vi "TCPIP.Server.vi"() -> ()   [LabVIEW 2011]
panel:
  out "Client Connected":bool
  out "Command (from Python)":string
  out "Return Value String (for Python)":string
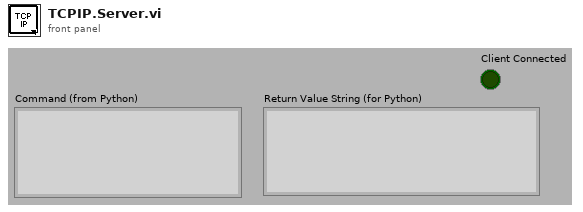
[diagram p1: front panel]
types:
  T1 = enum16{"Standard", "Buffered", "CRLF", "Immediate"}
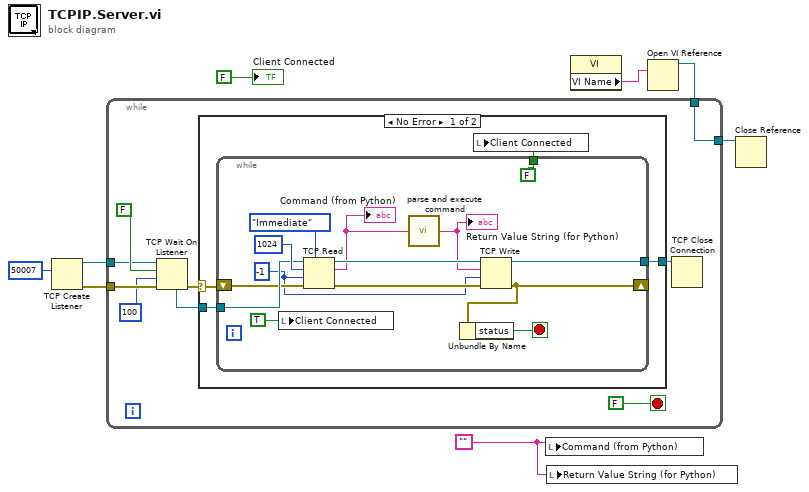
[diagram p0: block diagram]
diagram:
  w4 = ""
  n1 = TCP Create Listener(10:u16 50007 ("port")) -> (0:w8:errorcluster, 3:w1:refnum<k5>)  [unwired: 4 in, 1 out]
  n2 = local write "Command (from Python)"(w4) -> ()
  n3 = local write "Return Value String (for Python)"(w4) -> ()
  n4 = property class="VI"() -> ("VI Name"=w7:string)  [unwired: 2 in, 2 out]
  n5 = Open VI Reference(vi path=w7) -> (vi reference=w6:refnum<vi>)  [unwired: 5 in, 1 out]
  n6 = while {
    tunnel: w6 -> [w11]
    tunnel: [w11] -> w5
    tunnel: w8 -> [w17]
    tunnel: w1 -> [w9]
    stop <- FALSE stop-if-true
    n7 = TCP Wait On Listener(8:w17, 9:100 ("timeout ms (wait forever: -1)"), 10:FALSE ("resolve remote address (T)"), 11:w9) -> (0:w10:errorcluster, 4:w14:refnum<k5>)  [unwired: 3 out]
    n8 = case shown="No Error" w10 {
      selector: w10 -> [w19 _]
      tunnel: w14 -> [w21 w36]
      tunnel: [w20 w36] -> w13
      frame No Error {
        n9 = while {
          tunnel: [FALSE ("Connected")] -> w18
          shift-left: w19 -> [w30]
          shift-right: [w29] -> _
          tunnel: [w31] -> w20
          tunnel: w21 -> [w32]
          stop <- w22 stop-if-true
          w26 = -1 ("timeout ms (25000)")
          n10 = local write "Client Connected"(TRUE ("Connected")) -> ()
          n11 = TCP Read(connection ID=w32, bytes to read=1024, error in (no error)=w30, 7:T1."Immediate" ("mode (standard)"), 9:w26) -> (connection ID out=w25:refnum<k5>, data out=w23:string, error out=w33:errorcluster)
          "Command (from Python)" <- w23
          n12 = call "parse and execute command.vi"("Python Command"=w23) -> ("Python Return String"=w24:string)
          "Return Value String (for Python)" <- w24
          n13 = TCP Write(connection ID=w25, data in=w24, error in (no error)=w33, 9:w26) -> (connection ID out=w31:refnum<k5>, error out=w29:errorcluster)  [unwired: 1 out]
          n14 = Unbundle By Name(w29) -> ("status"=w22:bool)
        }
        n15 = local write "Client Connected"(w18) -> ()
      }
      frame Error {
      }
    }
    n16 = TCP Close Connection(connection ID=w13) -> ()  [unwired: 2 in, 2 out]
  }
  n17 = Close Reference(reference=w5) -> ()  [unwired: 1 in, 1 out]
  "Client Connected" <- FALSE ("Connected")
